vi "Get Display.vi"(8 "error in (no error)":errorcluster, 11 "VISA resource name":refnum<visa-resource-name>) -> (0 "error out":errorcluster, 1 "Channel":T1 items=["T0", "T1", "A", "B", "C", "D", "E", "F", "G", "H"], 2 "Display Value":i32(ring) items=["Trigger rate", "Trigger threshold", "Trigger single shot", "Trigger line", "Advanced triggering enable", "Trigger holdoff", "Prescale configuration", "Burst mode", "Burst delay", "Burst count", "Burst period", "Channel delay", "Channel output levels", "Channel output polarity", "Burst T0 configuration"], 3 "VISA resource name out":refnum<visa-resource-name>, 4 "Device Errors":cluster{"code":i32, "Text":string}[](array[cluster]))   [LabVIEW 2014, in "Stanford Research DG645 - Driver.lvlib"]
doc: "Status and Display Command: DISP?\nInstrument Error Check\n\nQuery the current display value i and the displayed channel c. The parameter i indicates the display type.\n\ni Display\n0 Trigger rate\n1 Trigger threshold\n2 Trigger single shot \n3 Trigger line\n4 Advanced triggering enable \n5 Trigger holdoff \n6 Prescale configuration\n7 Burst mode\n8 Burst delay\n8 Burst count\n10 Burst period \n11 Channel delay\n12 Channel output levels\n13 Channel output polarity\n14 Burst T0 configuration"
uses:
  Stanford Research DG645 - Driver.lvlib
  Channel.ctl
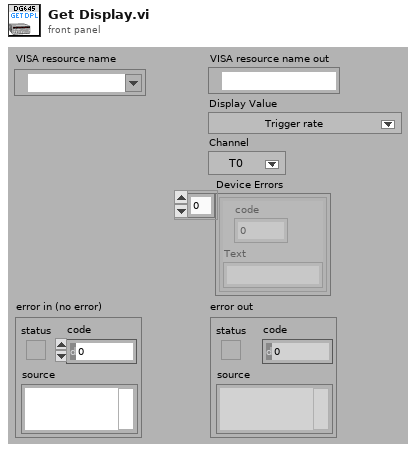
[diagram p1: front panel]
types:
  T1 = typedef "Stanford Research DG645 - Driver.lvlib/Channel.ctl" = i32
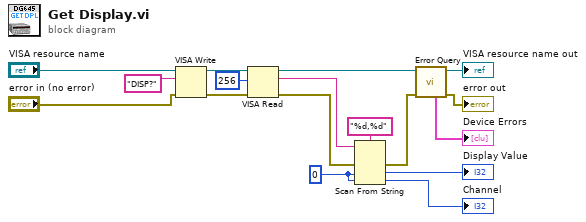
[diagram p0: block diagram]
diagram:
  w1 = 0 ("default value 1")
  n1 = VISA Write(VISA resource name="VISA resource name", write buffer="DISP?" ("command"), error in (no error)="error in (no error)") -> (VISA resource name out=w16:refnum<visa-resource-name>, error out=w15:errorcluster)  [unwired: 1 out]
  n2 = VISA Read(VISA resource name=w16, byte count=u32 256, error in (no error)=w15) -> (VISA resource name out=w4:refnum<visa-resource-name>, read buffer=w13:string, error out=w11:errorcluster)  [unwired: 1 out]
  n3 = Scan From String(format string="%d,%d", input string=w13, error in=w11, default 1=w1, default 2=w1) -> (error out=w6:errorcluster, output 1=→"Display Value":i32, output 2=→"Channel":i32)  [unwired: 1 in, 2 out]
  n4 = call "Error Query.vi"("error in (no error)"=w6, "VISA resource name"=w4) -> ("error out"=→"error out":errorcluster, "VISA resource name out"=→"VISA resource name out":refnum<visa-resource-name>, "Device Errors"=→"Device Errors":cluster{"code":i32, "Text":string}[])  [unwired: 7 in]
